vi "Get Subscribe Data.vi"(8 "error in (no error)":errorcluster, 11 "Topic Actor Subscribe Command in":refnum<class "Topic Actor Subscribe Command.lvclass">) -> (0 "error out":errorcluster, 1 "Message Transport Interface":refnum<class "Message Transport Interface.lvclass">, 2 "Subscriber Name":string, 3 "Topic Actor Subscribe Command out":refnum<class "Topic Actor Subscribe Command.lvclass">)   [LabVIEW 2016, in "Stream Mediator.lvlib" / "Topic Actor Subscribe Command.lvclass"]
doc: "--\nCopyright © 2017 Composed SystemsI All rights reserved.\n\nAuthor: Jon McBee <jon.mcbee@composed.io>\n\nThis library is provided \"AS IS\" ,WITHOUT WARRANTIES OR\nCONDITIONS OF ANY KIND, either express or implied.\n\nComposed Systems -- composed.io\n\nStream 0.0.1.1\nJon McBee - Composed Systems\nCopyright (c) 2017, Composed Systems"
uses:
  <userlib>/Composed Systems/Stream/Mediator/Classes/Topic Actor Subscribe Command/Topic Actor Subscribe Command.lvclass
  <userlib>/Composed Systems/Stream/Mediator/Classes/Message Transport Interface/Message Transport Interface.lvclass
  <userlib>/Composed Systems/Stream/Mediator/Classes/Topic Actor Subscribe Command/Topic Actor Subscribe Command.lvclass/Topic Actor Subscribe Command.ctl
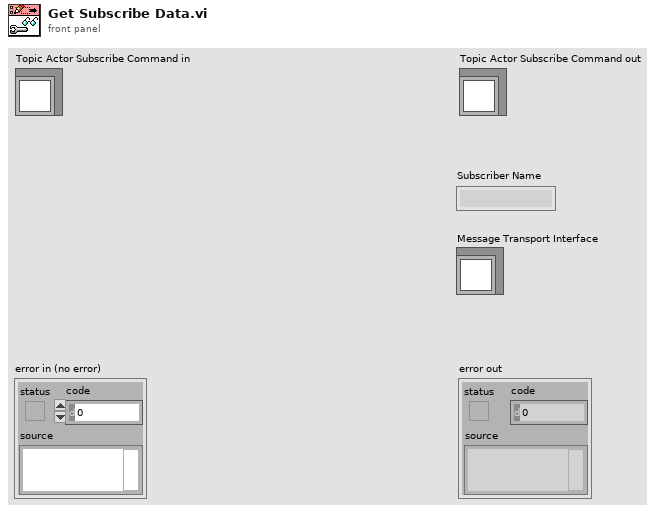
[diagram p1: front panel]
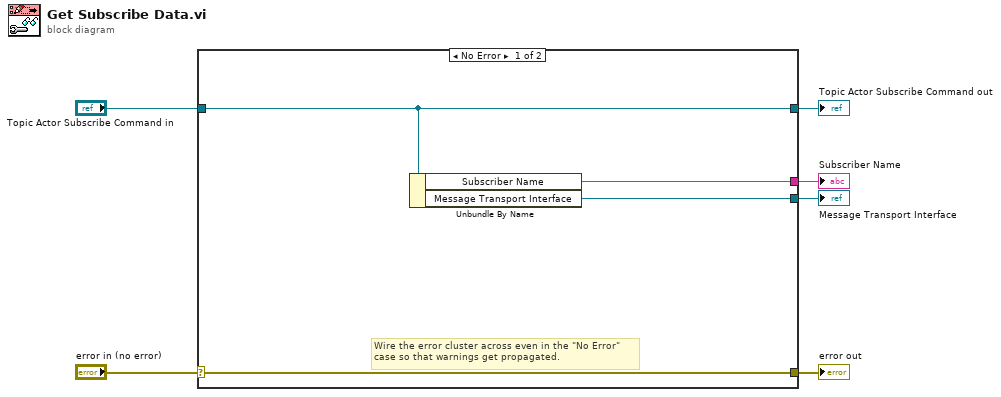
[diagram p0: block diagram]
diagram:
  n1 = case shown="No Error" "error in (no error)" {
    selector: "error in (no error)" -> [w10 w12]
    tunnel: [w10 w12] -> w5
    tunnel: [w9 w11] -> w3
    tunnel: "Topic Actor Subscribe Command in" -> [w9 w11]
    tunnel: [w8 _] -> w2
    tunnel: [w7 _] -> w1
    frame No Error {
      # "Wire the error cluster across even in the \"No Error\"\ncase so that warnings get propagated."
      n2 = Unbundle By Name(w9) -> ("Subscriber Name"=w8:string, "Message Transport Interface"=w7:refnum<class "Message Transport Interface.lvclass">)
    }
    frame Error {
    }
  }
  "error out" <- w5
  "Topic Actor Subscribe Command out" <- w3
  "Subscriber Name" <- w2
  "Message Transport Interface" <- w1
